vi "Actor Core.vi"(8 "error in":errorcluster, 11 "HIJ Vision Camera App In":refnum<class "HIJ Vision Camera App.lvclass">) -> (0 "error out":errorcluster, 3 "Actor out":refnum<class "Actor.lvclass">)   [LabVIEW 2020, in "HIJ Vision Camera App.lvlib" / "HIJ Vision Camera App.lvclass"]
doc: "(<B>Filename</B>: Actor Framework.lvlib:Actor.lvclass:Actor Core.vi)\n\nReceives messages to the actor, reacts to them, and initiates any error handling that may shut the actor down.\n\nDescendant classes may override this VI to append parallel tasks for the actor to complete while it handles messages. Overrides use the Call Parent Method node."
uses:
  HIJ Vision Camera App.lvclass
  C:/Program Files (x86)/National Instruments/LabVIEW 2020/vi.lib/ActorFramework/Actor/Actor.lvclass
  C:/Users/AlexK/work/LabVIEW Programme/POLARIS CAM Log Abw und E/Submodules/HIJ Vision/Application Base Actors/HIJ Vision Application/HIJ Vision Application/HIJ Vision Application.lvclass
  <vilib>/ActorFramework/Actor/Actor.lvclass
  HIJ Vision Camera App Messages/Camera Quick Settings Msg/Camera Quick Settings Msg.lvclass
  C:/Users/AlexK/work/LabVIEW Programme/POLARIS CAM Log Abw und E/Submodules/HIJ Vision/Display Actors/HIJ Vision Display/HIJ Vision Display Messages/Show or Hide Quick Settings Msg/Show or Hide Quick Settings Msg.lvclass
  <vilib>/ActorFramework/Actor/Actor.lvclass/Actor.ctl
  <vilib>/ActorFramework/Message Enqueuer/Message Enqueuer.lvclass/Message Enqueuer.ctl
  HIJ Vision Camera App.lvclass/HIJ Vision Camera App.ctl
  Display Actors/HIJ Vision Display/HIJ Vision Display Messages/Show or Hide Quick Settings Msg/Show or Hide Quick Settings Msg.lvclass/Show or Hide Quick Settings Msg.ctl
  HIJ Vision Application/HIJ Vision Application/HIJ Vision Application.lvclass/HIJ Vision Application.ctl
  Display Actors/HIJ Vision Display/HIJ Vision Display/HIJ Vision Display.lvclass/HIJ Vision Display.ctl
  HIJ Vision Camera App Messages/Write ConfigDir Msg/Write ConfigDir Msg.lvclass/Write ConfigDir Msg.ctl
  HIJ Vision Application/HIJ Vision Application Messages/Write Image Prefix Msg/Write Image Prefix Msg.lvclass/Write Image Prefix Msg.ctl
  HIJ Vision Camera App Messages/Start Aquisition Msg/Start Aquisition Msg.lvclass/Start Aquisition Msg.ctl
  Display Actors/HIJ Vision Display/HIJ Vision Display Messages/Show or Hide Quick Settings Msg/Write Caller Enqueuer.vi
  HIJ Vision Application/HIJ Vision Application/Read HIJ Vision Display.vi
  Read Overlay Font.vi
  Read Save Source in Filename.vi
  Read SaveTimestamp.vi
  Read TimestampFormat.vi
  Read ShotIdInFileName.vi
  Read FrameNrInFilename.vi
  HIJ Vision Application/HIJ Vision Application/Read ConfigDir.vi
  Display Actors/HIJ Vision Display/HIJ Vision Display/Write Overlay Font.vi
  Display Actors/HIJ Vision Display/HIJ Vision Display/Write Source in Filename.vi
  Display Actors/HIJ Vision Display/HIJ Vision Display/Write Time in Filename_.vi
  Display Actors/HIJ Vision Display/HIJ Vision Display/Write TimestampFormat.vi
  Display Actors/HIJ Vision Display/HIJ Vision Display/Write ShotId in Filename.vi
  Display Actors/HIJ Vision Display/HIJ Vision Display/Write FrameID in Filename.vi
  Display Actors/HIJ Vision Display/HIJ Vision Display/Write Show or Hide Quick Settings Msg.vi
  <vilib>/ActorFramework/Message Enqueuer/Init from Existing Queue.vi
  <vilib>/ActorFramework/Message Enqueuer/Enqueue.vi
  Camera Actors/Camera Actor/Camera Actor/Camera Actor.lvclass
  HIJ Vision Camera App Messages/Write ConfigDir Msg/Write ConfigDir Msg.lvclass
  C:/Program Files (x86)/National Instruments/LabVIEW 2020/vi.lib/ActorFramework/Message/Message.lvclass
  HIJ Vision Application/HIJ Vision Application Messages/Write Image Prefix Msg/Write Image Prefix Msg.lvclass
  HIJ Vision Camera App Messages/Start Aquisition Msg/Start Aquisition Msg.lvclass
  <vilib>/ActorFramework/Message Priority Queue/Priority Enqueue.vi
  HIJ Vision Application/HIJ Vision Application/Write HIJ Vision Display.vi
  <vilib>/ActorFramework/Message Enqueuer/Message Enqueuer.lvclass
  Display Actors/HIJ Vision Display/HIJ Vision Display/HIJ Vision Display.lvclass
  HIJ Vision Application/HIJ Vision Application/HIJ Vision Application.lvclass
  C:/Users/AlexK/work/LabVIEW Programme/POLARIS CAM Log Abw und E/Submodules/Viewable Actor/ViewableActor/ViewableActor.lvclass
  C:/Users/AlexK/work/LabVIEW Programme/POLARIS CAM Log Abw und E/Submodules/HIJ Vision/Analyze/Analyze Actor/IAnalysis/IAnalysis.lvclass
  C:/Users/AlexK/work/LabVIEW Programme/POLARIS CAM Log Abw und E/Submodules/HIJ Vision/Application Base Actors/HIJ Vision Camera App/HIJ Vision Camera App/HIJ Vision Camera App.lvclass
  C:/Users/AlexK/work/LabVIEW Programme/POLARIS CAM Log Abw und E/Submodules/HIJ Vision/Camera Actors/Camera Actor/ICamera/ICamera.lvclass
  C:/Users/AlexK/work/LabVIEW Programme/POLARIS CAM Log Abw und E/Submodules/HIJ Vision/Camera Actors/Camera Actor/Camera Actor/Camera Actor.lvclass
  C:/Users/AlexK/work/LabVIEW Programme/POLARIS CAM Log Abw und E/Submodules/HIJ Vision/Application Base Actors/HIJ Vision Camera App/HIJ Vision Camera App Messages/Camera Quick Settings Msg/Camera Quick Settings Msg.lvclass
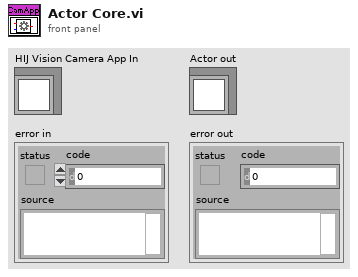
[diagram p1: front panel]
types:
  T1 = cluster{"Desired Font (Application)":enum16{"User-specified Font", "Application Font", "System Font", "Dialog Font"}, "[User-specified Font]":cluster{"Font Name":string, "Size":i16, "Strikeout?":bool, "Italic?":bool, "Underline?":bool, "Outline?":bool, "Shadow?":bool, "Bold?":bool, "Rotation Angle":dbl}, "Horizontal Alignment":i16, "Vertical Alignment":i16}
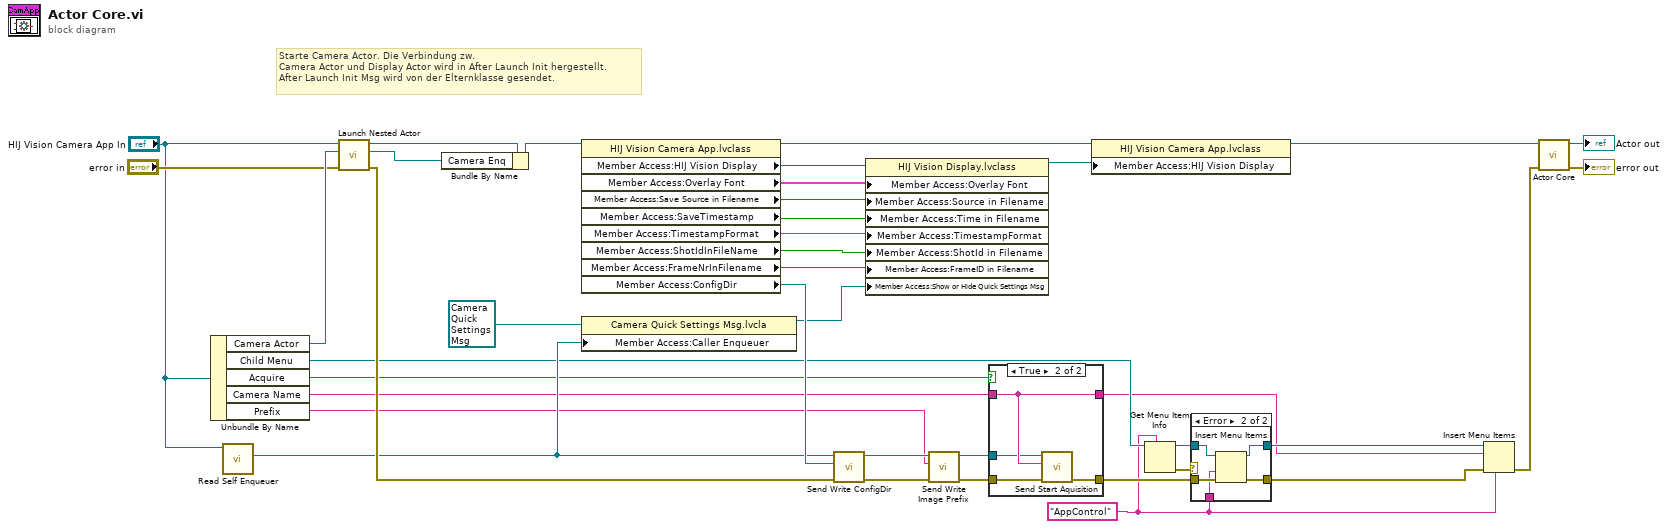
[diagram p0: block diagram]
diagram:
  w5 = "AppControl"
  # "Starte Camera Actor. Die Verbindung zw.\nCamera Actor und Display Actor wird in After Launch Init hergestellt.\nAfter Launch Init Msg wird von der Elternklasse gesendet."
  n1 = Unbundle By Name("HIJ Vision Camera App In") -> ("Camera Actor"=w37:refnum<class "Camera Actor.lvclass">, "Child Menu"=w35:refnum<k9>, "Acquire"=w11:bool, "Camera Name"=w10:string, "Prefix"=w3:string)
  n2 = call <vilib>:"Read Self Enqueuer.vi"("Actor"="HIJ Vision Camera App In") -> ("Self Enqueuer"=w36:refnum<class "Message Enqueuer.lvclass">)  [unwired: 10 in]
  n3 = call <vilib>:"Launch Nested Actor.vi"("error in (no error)"="error in", "Nested Actor"=w37, "Caller Actor in"="HIJ Vision Camera App In") -> ("error out"=w39:errorcluster, "Nested Actor's Enqueuer"=w31:refnum<class "Message Enqueuer.lvclass">, "Caller Actor out"=w20:refnum<class "HIJ Vision Camera App.lvclass">)  [unwired: 6 in]
  n4 = Bundle By Name(cluster=w20, "Camera Enq"=w31) -> (w24:refnum<class "HIJ Vision Camera App.lvclass">)
  n5 = property class="HIJ Vision Camera App.lvclass"(reference=w24) -> (reference out=w19:refnum<class "HIJ Vision Camera App.lvclass">, "Member Access:HIJ Vision Display"=w2:refnum<class "HIJ Vision Display.lvclass">, "Member Access:Overlay Font"=w17:T1, "Member Access:Save Source in Filename"=w16:bool, "Member Access:SaveTimestamp"=w15:bool, "Member Access:TimestampFormat"=w14:string, "Member Access:ShotIdInFileName"=w13:bool, "Member Access:FrameNrInFilename"=w12:bool, "Member Access:ConfigDir"=w38:path)  [unwired: 1 in, 1 out]
  n6 = property class="Camera Quick Settings Msg.lvcla"(reference=refnum<class "Camera Quick Settings Msg.lvclass"> refnum ("HIJ Vision Camera App.lvlib:Camera Quick Settings Msg.lvclass"), "Member Access:Caller Enqueuer"=w36) -> (reference out=w18:refnum<class "Camera Quick Settings Msg.lvclass">)  [unwired: 1 in, 1 out]
  n7 = call "Send Write ConfigDir.vi"("error in (no error)"=w39, "Work Dir"=w38, "Message Enqueuer"=w36) -> ("error out"=w28:errorcluster, "Message Enqueuer out"=w29:refnum<class "Message Enqueuer.lvclass">)  [unwired: 7 in]
  n8 = property class="HIJ Vision Display.lvclass"(reference=w2, "Member Access:Overlay Font"=w17, "Member Access:Source in Filename"=w16, "Member Access:Time in Filename"=w15, "Member Access:TimestampFormat"=w14, "Member Access:ShotId in Filename"=w13, "Member Access:FrameID in Filename"=w12, "Member Access:Show or Hide Quick Settings Msg"=w18) -> (reference out=w22:refnum<class "HIJ Vision Display.lvclass">)  [unwired: 1 in, 1 out]
  n9 = call "Send Write Image Prefix.vi"("error in (no error)"=w28, "Prefix"=w3, "Message Enqueuer"=w29) -> ("error out"=w26:errorcluster, "Message Enqueuer out"=w27:refnum<class "Message Enqueuer.lvclass">)  [unwired: 7 in]
  n10 = case shown="True" w11 {
    tunnel: w10 -> [w40 w45]
    tunnel: w27 -> [_ w44]
    tunnel: w26 -> [w41 w43]
    tunnel: [w41 w42] -> w25
    tunnel: [w40 w45] -> w1
    frame False {
    }
    frame True {
      n11 = call "Send Start Aquisition.vi"("error in (no error)"=w43, "Camera"=w45, "Message Enqueuer"=w44) -> ("error out"=w42:errorcluster)  [unwired: 7 in, 1 out]
    }
  }
  n12 = property class="HIJ Vision Camera App.lvclass"(reference=w19, "Member Access:HIJ Vision Display"=w22) -> (reference out=w23:refnum<class "HIJ Vision Camera App.lvclass">)  [unwired: 1 in, 1 out]
  n13 = Get Menu Item Info(7:w5, 11:w35) -> (0:w6:errorcluster, 3:w7:refnum<k9>)  [unwired: 1 in, 5 out]
  n14 = case shown="Error" w6 {
    tunnel: [w46 w52] -> w9
    tunnel: [w47 w51] -> w8
    tunnel: w7 -> [w47 w50]
    tunnel: w25 -> [w46 w49]
    tunnel: w5 -> [_ w48]
    frame No Error {
    }
    frame Error {
      n15 = Insert Menu Items(6:w49, 7:w48, 9:w50) -> (0:w52:errorcluster, 3:w51:refnum<k9>)  [unwired: 3 in, 1 out]
    }
  }
  n16 = Insert Menu Items(5:w5, 6:w9, 8:w1, 9:w8) -> (0:w30:errorcluster)  [unwired: 2 in, 2 out]
  n17 = call-parent "Actor Core.vi"("error in"=w30, "HIJ Vision Application in"=w23) -> ("error out"=→"error out":errorcluster, "Actor out"=→"Actor out":refnum<class "Actor.lvclass">)  [unwired: 8 in]
